vi "set_config_cluster.vi"(8 "error in (no error)":errorcluster, 10 "config cluster variant":variant, 11 "FPGAWrapperDL090211Galvo in":refnum<class "FPGAWrapperDL090211Galvo.lvclass">) -> (0 "error out":errorcluster, 3 "FPGAWrapperDL090211Galvo out":refnum<class "FPGAWrapperDL090211Galvo.lvclass">)   [LabVIEW 2010, in "FPGAWrapperDL090211Galvo.lvclass"]
uses:
  FPGAWrapperDL090211Galvo.lvclass
  FPGAWrapperDL090211Galvo.lvclass/FPGAWrapperDL090211Galvo.ctl
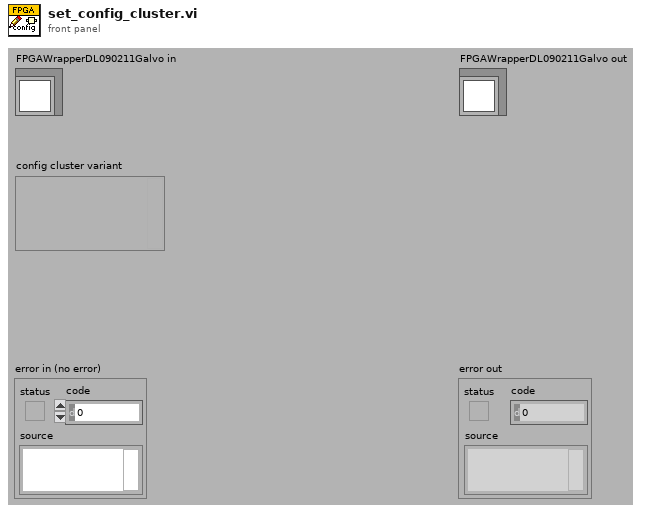
[diagram p1: front panel]
types:
  T1 = typedef "config_data_cluster.ctl" = cluster{"bit file":string, "hifo box version":i32, "ADC clock phase":i32}
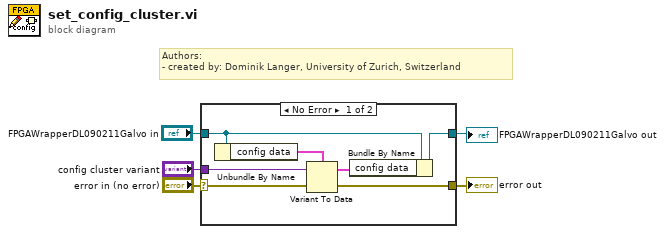
[diagram p0: block diagram]
diagram:
  # "Authors: \n- created by: Dominik Langer, University of Zurich, Switzerland"
  n1 = case shown="No Error" "error in (no error)" {
    selector: "error in (no error)" -> [w11 w13]
    tunnel: [w12 w13] -> w5
    tunnel: "FPGAWrapperDL090211Galvo in" -> [w10 w14]
    tunnel: [w9 w14] -> w2
    tunnel: "config cluster variant" -> [w6 _]
    frame No Error {
      n2 = Unbundle By Name(w10) -> ("config data"=w8:T1)
      n3 = Variant To Data(error in=w11, Variant=w6, type=w8) -> (error out=w12:errorcluster, data=w7:T1)
      n4 = Bundle By Name(cluster=w10, "config data"=w7) -> (w9:refnum<class "FPGAWrapperDL090211Galvo.lvclass">)
    }
    frame Error {
    }
  }
  "error out" <- w5
  "FPGAWrapperDL090211Galvo out" <- w2
